vi "Close LabVIEW.vi"(6 "User Event in":refnum<user-event>, 8 "error in (no error)":errorcluster) -> ()   [LabVIEW 2018]
uses:
  User Event - Stop/User Event - Stop.lvlib
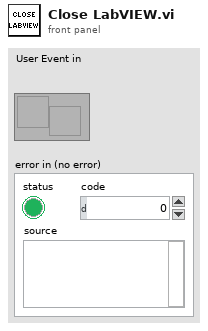
[diagram p1: front panel]
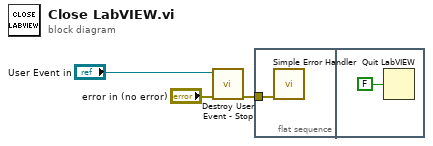
[diagram p0: block diagram]
diagram:
  n1 = call "Destroy User Event - Stop.vi"("error in (no error)"="error in (no error)", "User Event - Stop"="User Event in") -> ("error out"=w3:errorcluster)  [unwired: 9 in]
  n2 = flat-sequence {
    tunnel: w3 -> [w4]
    frame #0 {
      n3 = call <vilib>:"Simple Error Handler.vi"("error in (no error)"=w4) -> ()  [unwired: 4 in, 5 out]
    }
    frame #1 {
      n4 = Quit LabVIEW(quit? (T)=FALSE) -> ()
    }
  }
